vi "Get Image Delays.vi"(8 "error in (no error)":errorcluster, 11 "Save Image in":refnum<class "Save Image.lvclass">) -> (0 "error out":errorcluster, 3 "Save Image out":refnum<class "Save Image.lvclass">)   [LabVIEW 2018, in "Save Image.lvclass"]
uses:
  Save Image.lvclass
  Save Image.lvclass/Save Image.ctl
  Simulated_Header/Simulated_Header.lvclass
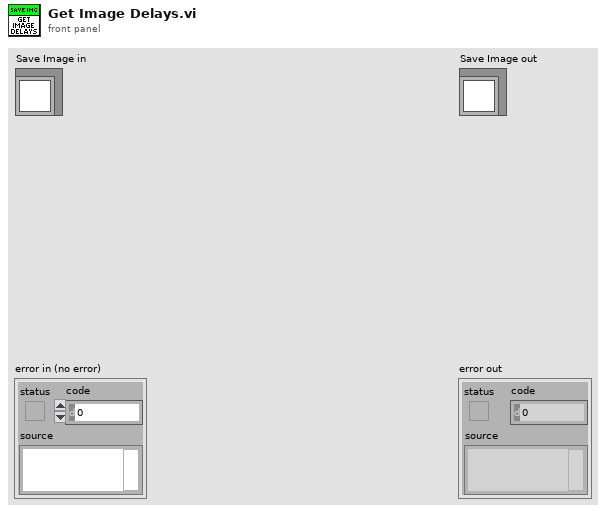
[diagram p1: front panel]
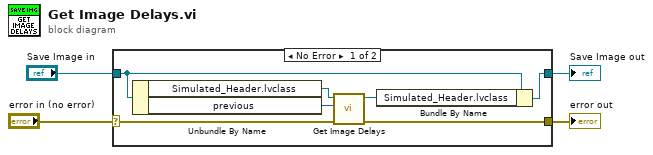
[diagram p0: block diagram]
diagram:
  n1 = case shown="No Error" "error in (no error)" {
    selector: "error in (no error)" -> [w10 w13]
    tunnel: [w6 w13] -> w3
    tunnel: [w5 w12] -> w1
    tunnel: "Save Image in" -> [w8 w12]
    frame No Error {
      n2 = Unbundle By Name(w8) -> ("Simulated_Header.lvclass"=w9:refnum<class "Simulated_Header.lvclass">, "previous"=w11:u16)
      n3 = call-dynamic "Get Image Delays.vi"("error in (no error)"=w10, "frames"=w11, "Simulated_Header in"=w9) -> ("error out"=w6:errorcluster, "Simulated_Header out"=w7:refnum<class "Simulated_Header.lvclass">)  [unwired: 7 in]
      n4 = Bundle By Name(cluster=w8, "Simulated_Header.lvclass"=w7) -> (w5:refnum<class "Save Image.lvclass">)
    }
    frame Error {
    }
  }
  "error out" <- w3
  "Save Image out" <- w1
